vi "Temperature Multiplot.vi"() -> ()   [LabVIEW 2010]
doc: "This VI is a solution to an exercise in the LabVIEW Core I course.\n\nThis VI acquires temperature values every 500 ms and also takes a running average of the last three temperature measurements and displays both the raw data and the running average in the strip chart."
panel:
  out "Temperature History":cluster{dbl, "Temperature":dbl}(graph)
  in  "Power":bool=TRUE
  # "ON\n\nOFF"
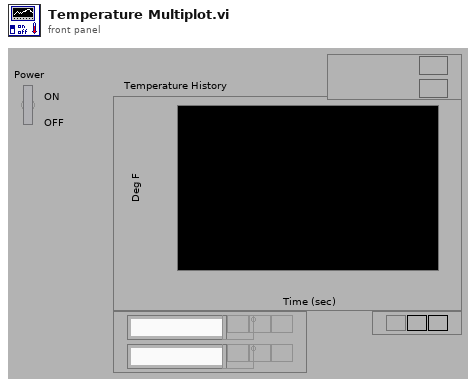
[diagram p1: front panel]
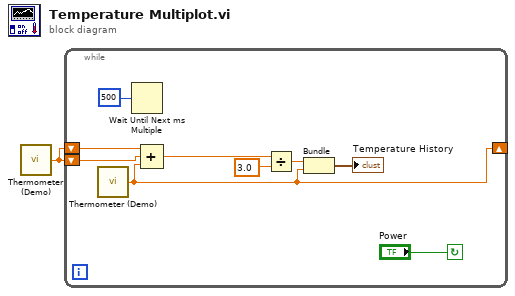
[diagram p0: block diagram]
diagram:
  n1 = call "Thermometer (Demo).vi"() -> ("Temperature"=w1:dbl)  [unwired: 1 in]
  n2 = while {
    shift-left: w1 -> [w7]
    shift-left: w1 -> [w8]
    shift-right: [w3] -> _
    stop <- "Power" continue-if-true
    n3 = call "Thermometer (Demo).vi"() -> ("Temperature"=w3:dbl)  [unwired: 1 in]
    n4 = Wait Until Next ms Multiple(millisecond multiple=u32 500) -> ()  [unwired: 1 out]
    n5 = Compound Arithmetic op=ADD(w8, w7, w3) -> (w6:dbl)
    n6 = Divide(x=w6, y=3.0 ("number: 0 to 1")) -> (x/y=w5:dbl)
    n7 = Bundle(w5, "Temperature"=w3) -> (→"Temperature History":cluster{dbl, "Temperature":dbl})  [unwired: 1 out]
  }
